vi "WPI_EncoderConfigureTimer.vi"(8 "error in (no error)":errorcluster, 9 "Number Samples to Average":u8=1 min=1 max=128, 10 "Minimum Rate":dbl=20.0, 11 "EncoderDevRef":T1={"DevStatus"={"status"=FALSE, "code"=0, "source"=""}, "EncoderIndex"=enum."Invalid", "CounterIndex"=enum."Ctr 1", "DistancePerCount"=2.0, "Decoding Type"=enum."4x"}) -> (0 "error out":errorcluster, 3 "EncoderDevRef":T1={"DevStatus"={"status"=FALSE, "code"=0, "source"=""}, "EncoderIndex"=enum."Invalid", "CounterIndex"=enum."Ctr 1", "DistancePerCount"=2.0, "Decoding Type"=enum."4x"})   [LabVIEW 2017]
doc: "Configures the timer for the encoder you specify. Use this VI to specify the minimum rate at which the CompactRIO device must receive pulses from the encoder before the device considers the encoder stopped. You also can use this VI to specify the number of samples of the timer to average when calculating the pulse rate. Use the Get VI to determine whether the encoder is stopped.\n\nThis software is licensed. Open the labview\\readme\\WPI Robotics Library Open Source License.txt file for more information."
uses:
  <vilib>/Rock Robotics/WPI/Encoder/WPI_EncoderDevRef.ctl
  <vilib>/Rock Robotics/SystemInterfaces/Encoder/FPGA_EncoderIdx.ctl
  <vilib>/Rock Robotics/SystemInterfaces/Counter/FPGA_CounterCtrSystemIndex.ctl
  <vilib>/Rock Robotics/WPI/Encoder/WPI_EncoderType.ctl
  <vilib>/Rock Robotics/SystemInterfaces/Encoder/FPGA_EncoderOpen WO Configuration.vi
  <vilib>/Rock Robotics/SystemInterfaces/Counter/FPGA_CounterERRInvalidResource.vi
  <vilib>/Rock Robotics/SystemInterfaces/Encoder/FPGA_EncoderERRInvalidResource.vi
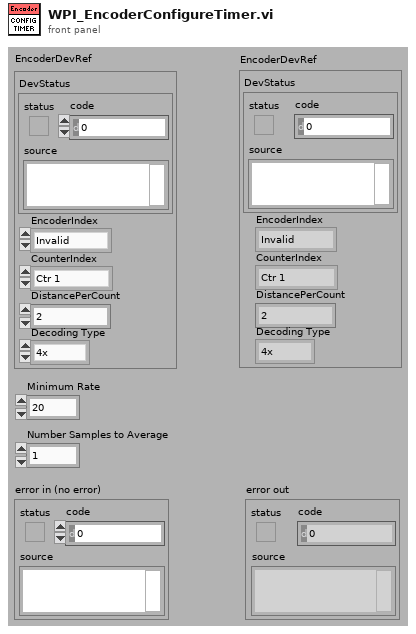
[diagram p1: front panel]
types:
  T1 = typedef "WPI_EncoderDevRef.ctl" = cluster{"DevStatus":errorcluster, "EncoderIndex":T2, "CounterIndex":T3, "DistancePerCount":dbl, "Decoding Type":T4}
  T2 = typedef "FPGA_EncoderIdx.ctl" = enum8{"Enc 0", "Enc 1", "Enc 2", "Enc 3", "Enc 4", "Enc 5", "Enc 6", "Enc 7", "Invalid"}
  T3 = typedef "FPGA_CounterCtrSystemIndex.ctl" = enum8{"Ctr 0", "Ctr 1", "Ctr 2", "Ctr 3", "Ctr 4", "Ctr 5", "Ctr 6", "Ctr 7", "Invalid"}
  T4 = typedef "WPI_EncoderType.ctl" = enum16{"1x", "2x", "4x"}
  T5 = typedef "FPGA_CounterCtrDevRef.ctl" = cluster{"DevStatus":errorcluster, "CntIndex":T3}
  T6 = typedef "FPGA_EncoderDevRef.ctl" = cluster{"EncoderIndex":T2, "DevStatus":errorcluster}
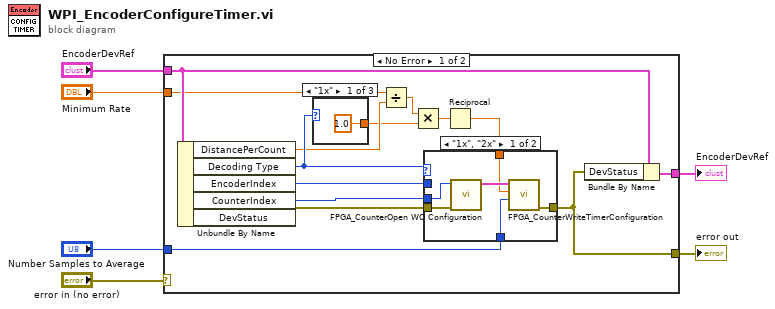
[diagram p0: block diagram]
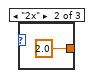
[diagram p2: hidden frame]
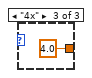
[diagram p3: hidden frame]
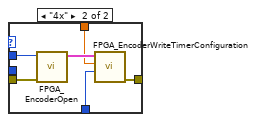
[diagram p4: hidden frame]
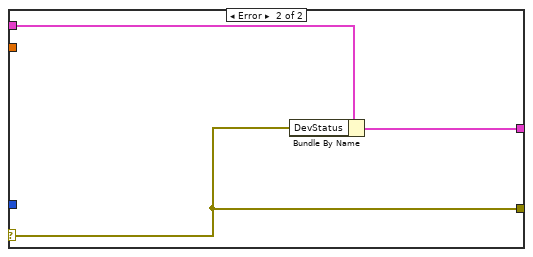
[diagram p5: hidden frame]
diagram:
  n1 = case shown="No Error" "error in (no error)" {
    selector: "error in (no error)" -> [_ w36]
    tunnel: "Minimum Rate" -> [w12 _]
    tunnel: "EncoderDevRef" -> [w17 w38]
    tunnel: [w20 w37] -> w5
    tunnel: [w15 w36] -> w3
    tunnel: "Number Samples to Average" -> [w14 _]
    frame No Error {
      n2 = Unbundle By Name(w17) -> ("DistancePerCount"=w8:dbl, "Decoding Type"=w13:T4, "EncoderIndex"=w18:T2, "CounterIndex"=w16:T3, "DevStatus"=w19:errorcluster)
      n3 = case shown="\"1x\"" w13 {
        tunnel: [1.0 2.0 4.0] -> w7
        frame "1x" {
        }
        frame "2x" {
        }
        frame "4x" {
        }
      }
      n4 = Divide(x=w12, y=w8) -> (x/y=w11:dbl)
      n5 = Multiply(x=w11, y=w7) -> (x*y=w10:dbl)
      n6 = Reciprocal(x=w10) -> (1/x=w9:dbl)
      n7 = case shown="\"1x\", \"2x\"" w13 {
        tunnel: w19 -> [w28 w35]
        tunnel: w18 -> [_ w34]
        tunnel: w9 -> [w25 w32]
        tunnel: [w29 w31] -> w15
        tunnel: w16 -> [w27 _]
        tunnel: w14 -> [w24 w30]
        frame "1x", "2x" {
          n8 = call <vilib>:"FPGA_CounterOpen WO Configuration.vi"("error in"=w28, "CntIndex"=w27) -> ("Ctr Ref"=w26:T5)  [unwired: 1 in, 8 out]
          n9 = call <vilib>:"FPGA_CounterWriteTimerConfiguration.vi"("Average Size"=w24, "StallPeriod (s)"=w25, "Ctr Ref in"=w26) -> ("error out"=w29:errorcluster)  [unwired: 2 in, 6 out]
        }
        frame "4x" {
          n10 = call-poly <vilib>:"FPGA_EncoderOpen.vi"("DeviceStatus"=w35, "EncoderIndex"=w34) -> ("Encoder Reference"=w33:T6)  [unwired: 1 in, 8 out]
          n11 = call <vilib>:"FPGA_EncoderWriteTimerConfiguration.vi"("AverageSize"=w30, "StallPeriod (sec)"=w32, "EncoderDevRef"=w33) -> ("error out"=w31:errorcluster)  [unwired: 1 in, 7 out]
        }
      }
      n12 = Bundle By Name(cluster=w17, "DevStatus"=w15) -> (w20:T1)
    }
    frame Error {
      n13 = Bundle By Name(cluster=w38, "DevStatus"=w36) -> (w37:T1)
    }
  }
  "EncoderDevRef" <- w5
  "error out" <- w3
